vi "Test Publish Folder Naming.vi"() -> ()   [LabVIEW 2010]
panel:
  out "drop location (new)":string
  in  "Folder":string="esvrs11"
  out "drop location":string
  in  "Site":string="ICE1"
  in  "Server":string="esvrs11"
  # "ICE1"
  # "esvrs11"
  # "icela_esvrs11\\BIMS\\File Drops\\ICE1"
  # "\\\\esvrs11\\icela_esvrs11\\BIMS\\File Drops\\ICE1\\ICE1.mdb"
  # "SPR1"
  # "sprs68"
  # "SP-BIMS-Filedrop$"
  # "\\\\sprs68\\SP-BIMS-Filedrop$\\SPR1.mdb"
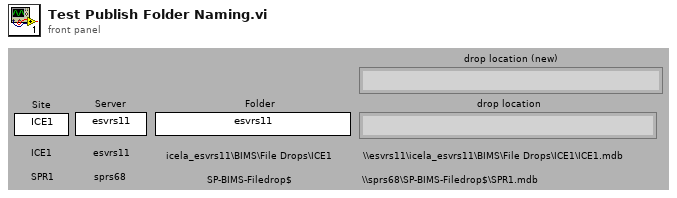
[diagram p1: front panel]
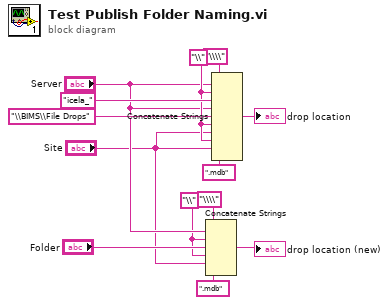
[diagram p0: block diagram]
diagram:
  w4 = "\\" ("string")
  w12 = "\\" ("string")
  n1 = Concatenate Strings("\\\\" ("string"), "Server", w4, "Folder", w4, "Site", ".mdb" ("string")) -> (→"drop location (new)":string)
  n2 = Concatenate Strings("\\\\" ("string"), "Server", w12, "icela_" ("string"), "Server", "\\BIMS\\File Drops" ("string"), w12, "Site", w12, "Site", ".mdb" ("string")) -> (→"drop location":string)
